vi "SMBus Write Byte.vi"(5 "PEC":u8, 6 "Data":u8, 7 "SlaveAddr":u8, 8 "error in (no error)":errorcluster, 9 "SMBUSIndex":i32, 10 "DevIndex":i32, 11 "DevType":i32) -> (0 "error out":errorcluster, 3 "function return":i32)   [LabVIEW 2012, in "ControlSMBus.lvlib"]
doc: "int WINAPI SMBus_WriteByte(int DevType,int DevIndex,int SMBUSIndex,unsigned char SlaveAddr,unsigned char Data,unsigned char PEC);"
uses:
  ControlSMBus.lvlib
  Ginkgo_Driver.dll
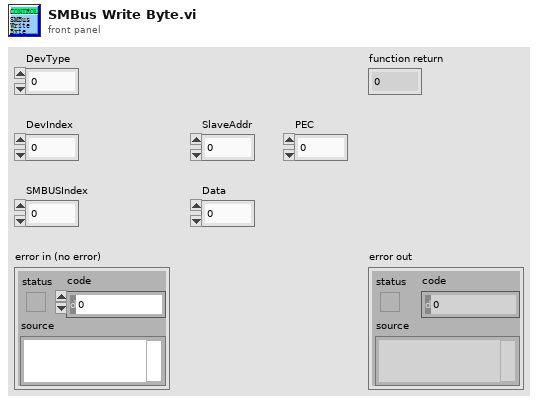
[diagram p1: front panel]
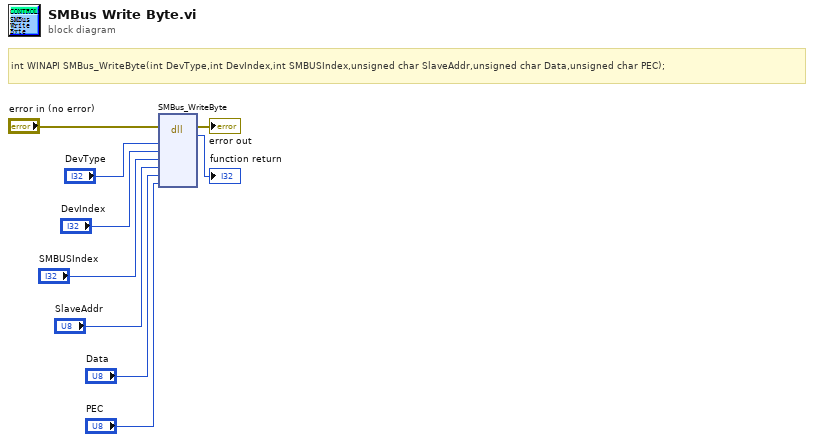
[diagram p0: block diagram]
diagram:
  # "int WINAPI SMBus_WriteByte(int DevType,int DevIndex,int SMBUSIndex,unsigned char SlaveAddr,unsigned char Data,unsigned char PEC);"
  n1 = dll-call lib="E:/Project/vt_ginkgo/truck/Ginkgo Driver/vs2010/Ginkgo_USB-I2C_API_v2.0.3.0/lib/labview_64bit/ControlSMBus/Ginkgo_Driver.*" fn="SMBus_WriteByte"(error in="error in (no error)", "DevType"="DevType", "DevIndex"="DevIndex", "SMBUSIndex"="SMBUSIndex", "SlaveAddr"="SlaveAddr", "Data"="Data", "PEC"="PEC") -> (error out=→"error out":errorcluster, →"function return":i32)  [unwired: 8 in, 1 out]
